vi "XY Graph Get Label.vi"(2 "XYGraph":refnum<vi>) -> (7 "Graph Label":string)   [LabVIEW 2019]
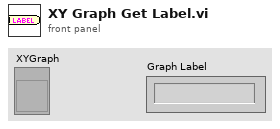
[diagram p1: front panel]
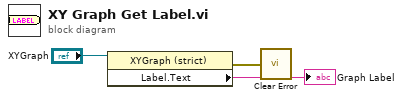
[diagram p0: block diagram]
diagram:
  n1 = property class="XYGraph (strict)"(reference="XYGraph") -> (error out=w1:errorcluster, "Label.Text"=→"Graph Label":string)  [unwired: 1 in, 1 out]
  n2 = call "Clear Error.vi"("Error In"=w1) -> ()  [unwired: 8 in, 1 out]
